vi "FUncionmatch.vi"(11 "Entrada":string="1:2023;1:1038;") -> (1 "Salida":string, 2 "number 2":i32, 3 "number":i32)   [LabVIEW 2023]
panel:
  out "String":string
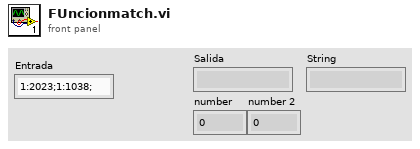
[diagram p1: front panel]
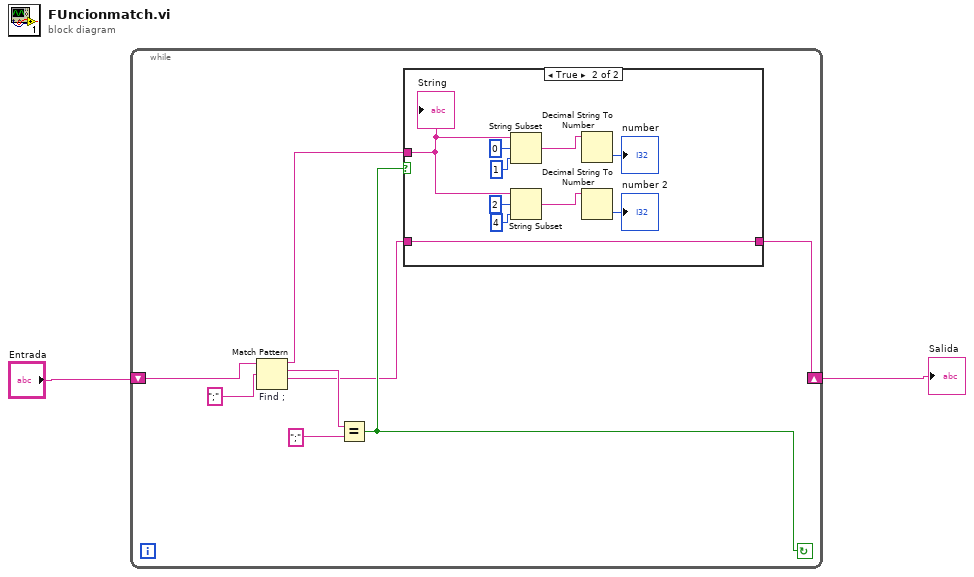
[diagram p0: block diagram]
diagram:
  n1 = while {
    shift-right: [w3] -> w2
    shift-left: "Entrada" -> [w10]
    stop <- w6 continue-if-true
    n2 = Match Pattern "Find ;"(string=w10, regular expression=";") -> (before substring=w5:string, match substring=w7:string, after substring=w4:string)  [unwired: 1 in, 1 out]
    n3 = Equal?(x=w7, y=";") -> (x = y?=w6:bool)
    n4 = case shown="True" w6 {
      tunnel: w5 -> [w11 w20]
      tunnel: w4 -> [_ w21]
      tunnel: [w11 w21] -> w3
      frame False {
      }
      frame True {
        n5 = String Subset(string=w20, offset (0)=0, length (rest)=1 ("length (rest)")) -> (substring=w17:string)
        n6 = String Subset(string=w20, offset (0)=2, length (rest)=4 ("length (rest)")) -> (substring=w16:string)
        n7 = Decimal String To Number(string=w17) -> (number=→"number":i32)  [unwired: 2 in, 1 out]
        n8 = Decimal String To Number(string=w16) -> (number=→"number 2":i32)  [unwired: 2 in, 1 out]
        "String" <- w20
      }
    }
  }
  "Salida" <- w2
